vi "Run Javascript.vi"(0 "Display State In":T1, 1 "Fetch Result":bool=TRUE, 5 "javaScript":string, 7 "Decode Result":bool=TRUE, 9 "Container State":T2, 11 "error in (no error)":errorcluster) -> (4 "Display State Out":T1, 6 "Result":string, 15 "error out":errorcluster)   [LabVIEW 2020, in "WebView2 XControl.lvlib" / "WebView2 Control.xctl"]
uses:
  WebView2 Control.xctl
  <vilib>/_xctls/Container State.ctl
  State.ctl
  Webview2 Lib/WebView2 Control Object/WebView2 Control.lvclass
  <vilib>/_xctls/XControlSupport.lvlib
panel:
  # "Add Controls & Indicators that form the parameters of the method here. Hook them to the connector pane. Do not delete the controls & indicators that are already hooked to the connector pane.\n \nTo setup the parameters  for this method, right click on this item in the Project Tree & select \"Configure Method...\"."
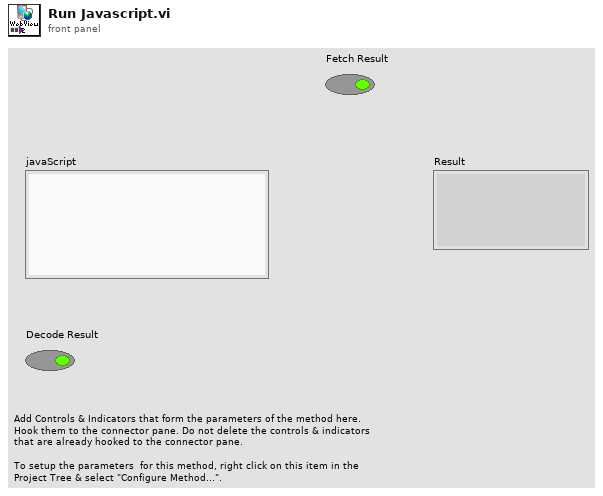
[diagram p1: front panel]
types:
  T1 = typedef "WebView2 XControl.lvlib/WebView2 Control.xctl/State.ctl" = cluster{"Control Object Ref":refnum<data-value>}
  T2 = typedef "XControlSupport.lvlib/Container State.ctl" = cluster{"Indicator?":bool, "Run Mode?":bool, " Refnum":refnum<vi>}
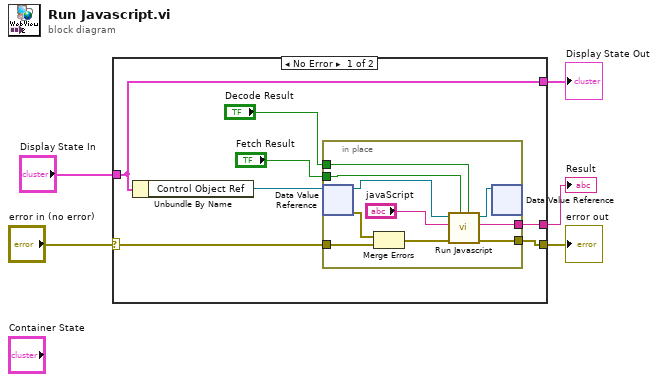
[diagram p0: block diagram]
diagram:
  n1 = case shown="No Error" "error in (no error)" {
    selector: "error in (no error)" -> [w7 w24]
    tunnel: [w8 w24] -> w4
    tunnel: "Display State In" -> [w12 w23]
    tunnel: [w12 w23] -> w2
    tunnel: [w6 _] -> w1
    frame No Error {
      n2 = Unbundle By Name(w12) -> ("Control Object Ref"=w11:refnum<data-value>)
      n3 = in-place {
        in-place-border: "Fetch Result" -> [w20]
        in-place-border: "Decode Result" -> [w19]
        in-place-border: [w16] -> w8
        in-place-border: w7 -> [w14]
        in-place-border: [w13] -> w6
        n4 = in-place-dvr #1(w11) -> (w22:refnum<class "WebView2 Control.lvclass">, w17:errorcluster)
        n5 = Merge Errors(w17, w14) -> (w15:errorcluster)
        n6 = call "Run Javascript.vi"("Decode Result (T)"=w19, "Fetch Result (T)"=w20, "error in (no error)"=w15, "javaScript"="javaScript", "WebView2 Control in"=w22) -> ("error out"=w16:errorcluster, "Result"=w13:string, "WebView2 Control out"=w21:refnum<class "WebView2 Control.lvclass">)  [unwired: 4 in]
        n7 = in-place-dvr #1(w21) -> ()  [unwired: 2 out]
      }
    }
    frame Error {
    }
  }
  "Display State Out" <- w2
  "error out" <- w4
  "Result" <- w1
